vi "Handle getAll.vi"(8 "error in (no error)":errorcluster, 11 "Inst.FP in":refnum<class "Inst.FP.lvclass">) -> (0 "error out":errorcluster, 2 "getAll":variant, 3 "Inst.FP out":refnum<class "Inst.FP.lvclass">)   [LabVIEW 2019, in "Inst.FP.lvclass"]
uses:
  Inst.FP.lvclass
  Inst.FP.lvclass/Inst.FP.ctl
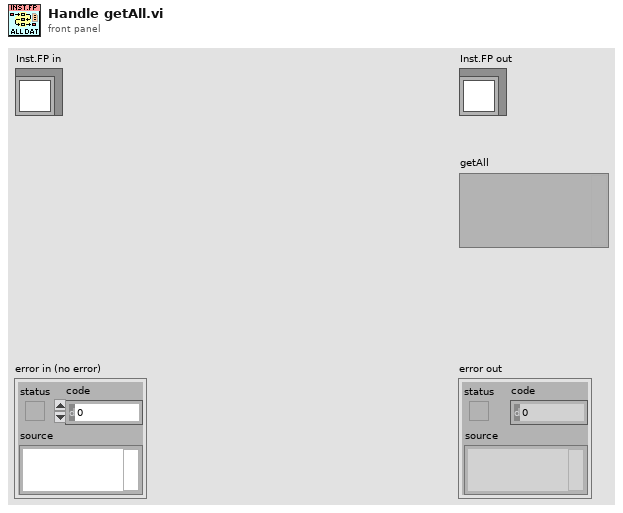
[diagram p1: front panel]
types:
  T1 = typedef "Inst.FP.lvclass/Inst.FP.getAll--Cluster.ctl" = cluster{"FP Data":dbl[], "MG Data":dbl[], "PT Data":dbl[], "Status Array":u32[], "Mode":string}
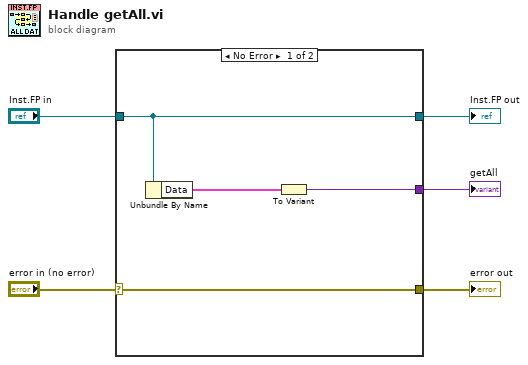
[diagram p0: block diagram]
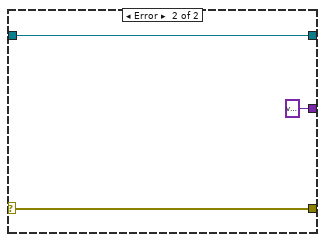
[diagram p2: hidden frame]
diagram:
  n1 = case shown="No Error" "error in (no error)" {
    selector: "error in (no error)" -> [w7 w11]
    tunnel: "Inst.FP in" -> [w8 w12]
    tunnel: [w6 variant ("Variant")] -> w4
    tunnel: [w8 w12] -> w2
    tunnel: [w7 w11] -> w1
    frame No Error {
      n2 = Unbundle By Name(w8) -> ("Data"=w9:T1)
      n3 = To Variant(anything=w9) -> (Variant=w6:variant)
    }
    frame Error {
    }
  }
  "error out" <- w1
  "Inst.FP out" <- w2
  "getAll" <- w4
